vi "Read Array.vi"(8 "error in (no error)":errorcluster, 11 "Test Properties in":refnum<class "Test Properties.lvclass">) -> (0 "error out":errorcluster, 2 "Array":u16[](array[ring]) items=["dev1", "5051"], 3 "Test Properties out":refnum<class "Test Properties.lvclass">)   [LabVIEW 2015, in "Test Properties.lvclass"]
uses:
  Test Properties.lvclass
  Test Properties.lvclass/Test Properties.ctl
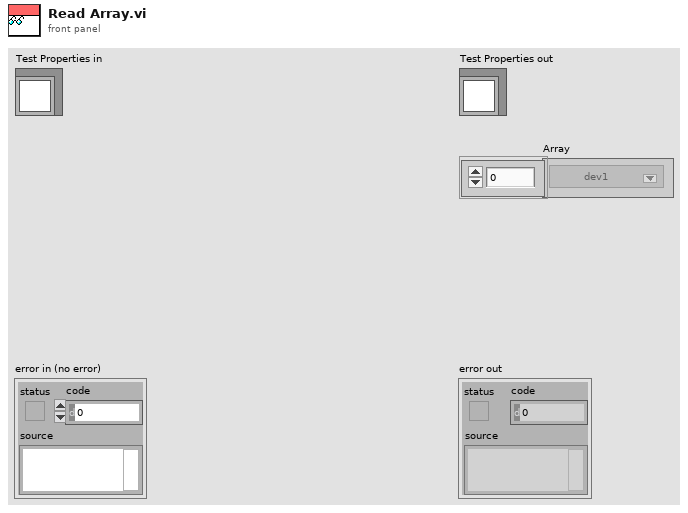
[diagram p1: front panel]
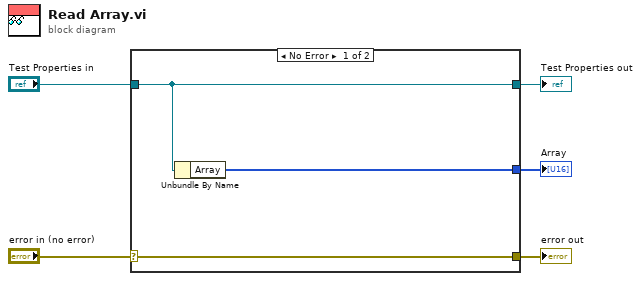
[diagram p0: block diagram]
diagram:
  n1 = case shown="No Error" "error in (no error)" {
    selector: "error in (no error)" -> [w8 w9]
    tunnel: [w8 w9] -> w4
    tunnel: [w7 w10] -> w2
    tunnel: "Test Properties in" -> [w7 w10]
    tunnel: [w6 _] -> w1
    frame No Error {
      n2 = Unbundle By Name(w7) -> ("Array"=w6:u16[])
    }
    frame Error {
    }
  }
  "error out" <- w4
  "Test Properties out" <- w2
  "Array" <- w1
